vi "Enqueue--update_complete_tour_text_indicator.vi"(8 "error in (no error)":errorcluster, 10 "tour number":u64, 11 "Completed tour paragraph":string) -> (0 "error out":errorcluster)   [LabVIEW 2020, in "main.lvlib"]
doc: "Blank VI with error handling."
uses:
  main.lvlib
  update_completed_tour_text_indicator arguments.ctl
panel:
  # "Development\ncontrols/indicators useful for development and testing, but which are not outputs of the VI"
  # "Input\nInputs to the VI"
  # "Output\nOutputs of the VI"
  # "Description\n\nBlank VI with error handling case. \n\nSummarize the use of this VI in this space."
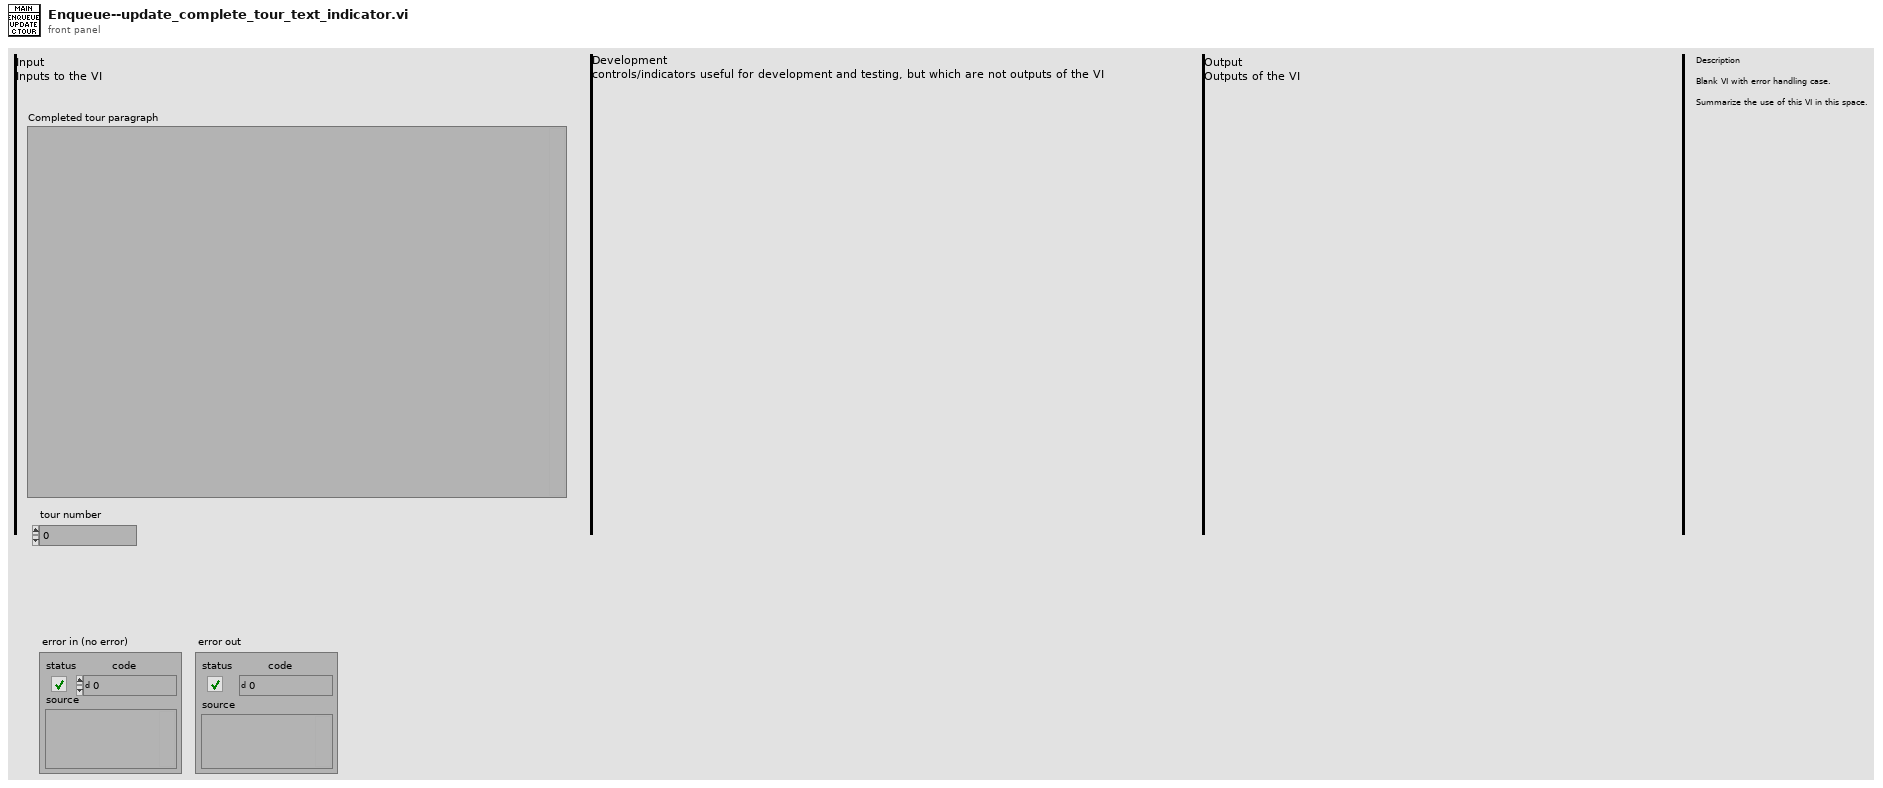
[diagram p1: front panel]
types:
  T1 = typedef "main.lvlib/update_completed_tour_text_indicator arguments.ctl" = cluster{"Completed tour paragraph":string, "tour number":u64}
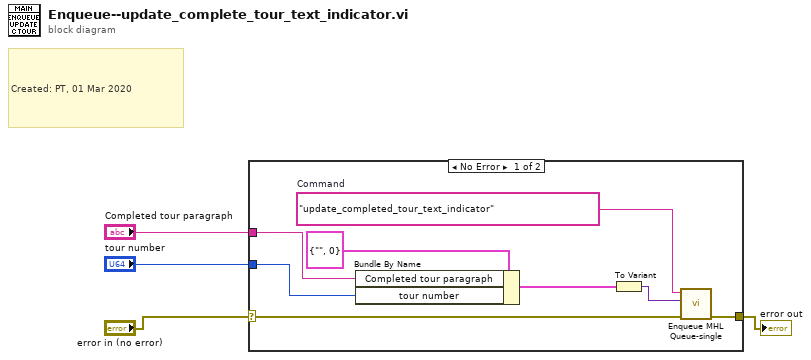
[diagram p0: block diagram]
diagram:
  # "Created: PT, 01 Mar 2020"
  n1 = case shown="No Error" "error in (no error)" {
    selector: "error in (no error)" -> [w11 w13]
    tunnel: [w10 w13] -> w3
    tunnel: "tour number" -> [w6 _]
    tunnel: "Completed tour paragraph" -> [w5 _]
    frame No Error {
      w12 = "update_completed_tour_text_indicator"  # Command
      n2 = Bundle By Name(cluster=T1 {"Completed tour paragraph"="", "tour number"=0} ("update_completed_tour_text_indicator arguments"), "Completed tour paragraph"=w5, "tour number"=w6) -> (w8:T1)
      n3 = To Variant(anything=w8) -> (Variant=w9:variant)
      n4 = call "Enqueue MHL Queue-single.vi"("ErrorIn"=w11, "Data"=w9, "Command"=w12) -> ("ErrorOut"=w10:errorcluster)  [unwired: 8 in]
    }
    frame Error {
    }
  }
  "error out" <- w3
